vi "StahlPS_Pbus.UpdateOnOff.vi"(0 "i ref in":refnum<vi>, 1 "badValue":bool, 2 "moduleValue":dbl format="%.2f", 3 "ms timeout (10000)":i32=10000, 5 "error in (no error)":errorcluster, 6 "onOffQuality":i32) -> (14 "i ref out":refnum<vi>, 17 "timed out":bool, 19 "error out":errorcluster)   [LabVIEW 2014, in "StahlPS_Pbus.lvlib"]
doc: "Takes the value published by the module and calculates the on-off state.\n\nThe value is written to the attribute data and published via DIM.\n\nThe bad-status bit is also determined and updated."
uses:
  StahlPS_Pbus.lvlib
  CSlibraries/UtilityLib/UtilityLib.valueStatus.ctl
  CSCore/CSApplicationBaseClasses/PSChannelBase/PSChannelBase.statusType.ctl
  CSCore/CSApplicationBaseClasses/PSChannelBase/PSChannelBase.directionType.ctl
  CSCore/CSApplicationBaseClasses/PSChannelBase/PSChannelBase.serviceType.ctl
  CSCore/CSApplicationBaseClasses/DeviceBase/DeviceBase.deviceState.ctl
  CSCore/CSApplicationBaseClasses/PSChannelBase/PSChannelBase.lvlib
  CSlibraries/UtilityLib/UtilityLib.lvlib
  CSCore/CSApplicationBaseClasses/DeviceBase/DeviceBase.lvlib
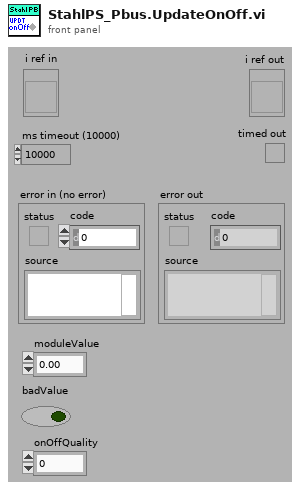
[diagram p1: front panel]
types:
  T1 = typedef "UtilityLib.lvlib/UtilityLib.valueStatus.ctl" = enum16{"no info available", "stand by/off", "on", "warning", "alarm/malfunction", "not implemented", "user action required", "important information", "system default", "control default", "indicator default", "button default"}
  T2 = typedef "PSChannelBase.lvlib/PSChannelBase.serviceType.ctl" = enum16{"onOff", "voltage", "current", "tripCurrent", "rampUpSpeed", "rampDownSpeed", "status"}
  T3 = typedef "DeviceBase.lvlib/DeviceBase.deviceState.ctl" = i16
  T4 = typedef "PSChannelBase.lvlib/PSChannelBase.directionType.ctl" = enum16{"unknown", "update actual value", "update nominal value", "update both"}
  T5 = typedef "PSChannelBase.lvlib/PSChannelBase.statusType.ctl" = i32
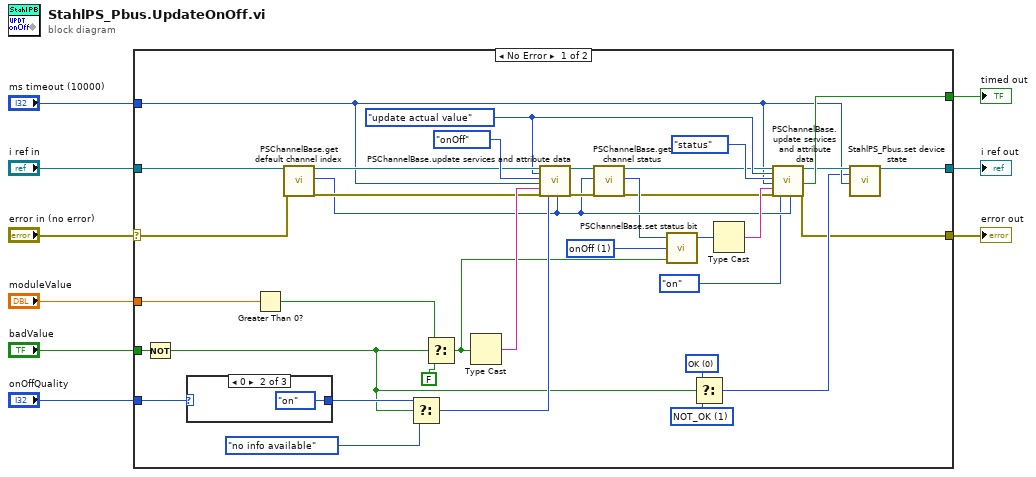
[diagram p0: block diagram]
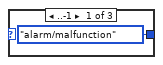
[diagram p2: hidden frame]
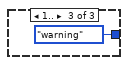
[diagram p3: hidden frame]
diagram:
  n1 = case shown="No Error" "error in (no error)" {
    selector: "error in (no error)" -> [w29 w49]
    tunnel: "i ref in" -> [w30 w50]
    tunnel: "moduleValue" -> [w32 _]
    tunnel: "ms timeout (10000)" -> [w15 _]
    tunnel: [w16 w50] -> w6
    tunnel: [w10 w49] -> w5
    tunnel: [w33 _] -> w4
    tunnel: "badValue" -> [w45 _]
    tunnel: "onOffQuality" -> [w44 _]
    frame No Error {
      w14 = T3 1 items=["ERROR"=-1, "OK"=0, "NOT_OK"=1] ("f")
      w13 = T3 0 items=["ERROR"=-1, "OK"=0, "NOT_OK"=1] ("deviceState")
      w37 = PSChannelBase.directionType."update actual value" ("direction")
      w24 = T5 1 items=["onOff"=1, "inRange"=2, "rampingUp"=4, "rampingDown"=8, "tripped"=16, "error"=32] ("service")
      n2 = Not(x=w45) -> (.not. x?=w12:bool)
      n3 = case shown="0" w44 {
        tunnel: [UtilityLib.valueStatus."alarm/malfunction" ("quality") UtilityLib.valueStatus."on" ("quality") UtilityLib.valueStatus."warning" ("quality")] -> w43
        frame ..-1 {
        }
        frame 0 {
        }
        frame 1.. {
        }
      }
      n4 = Greater Than 0?(x=w32) -> (x > 0?=w23:bool)
      n5 = call "PSChannelBase.get default channel index.vi"("i ref in"=w30, "error in (no error)"=w29) -> ("i ref out"=w39:refnum<vi>, "defaultChannelIndex"=w26:i32, "error out"=w38:errorcluster)  [unwired: 15 in]
      n6 = Select(t=w43, s=w12, f=UtilityLib.valueStatus."no info available" ("quality")) -> (s? t:f=w35:T1)
      n7 = Select(t=w23, s=w12, f=FALSE) -> (s? t:f=w18:bool)
      n8 = Type Cast(x=w18) -> (*(type *) &x=w40:string)  [unwired: 1 in]
      n9 = call "PSChannelBase.update services and attribute data.vi"("i ref in"=w39, "direction"=w37, "service"=PSChannelBase.serviceType."onOff", "ms timeout (10000)"=w15, "value"=w40, "error in (no error)"=w38, "quality"=w35, "channelNumber"=w26) -> ("i ref out"=w28:refnum<vi>, "error out"=w27:errorcluster)  [unwired: 9 in, 1 out]
      n10 = call "PSChannelBase.get channel status.vi"("i ref in"=w28, "channelIndex"=w26, "error in (no error)"=w27) -> ("i ref out"=w20:refnum<vi>, "status"=w25:i32, "error out"=w19:errorcluster)  [unwired: 14 in]
      n11 = call "PSChannelBase.set status bit.vi"("set"=w18, "statusBit"=w24, "status"=w25) -> ("status out"=w22:T5)  [unwired: 2 in]
      n12 = Select(t=w13, s=w12, f=w14) -> (s? t:f=w11:T3)
      n13 = Type Cast(x=w22) -> (*(type *) &x=w34:string)  [unwired: 1 in]
      n14 = call "PSChannelBase.update services and attribute data.vi"("i ref in"=w20, "direction"=w37, "service"=PSChannelBase.serviceType."status", "ms timeout (10000)"=w15, "value"=w34, "error in (no error)"=w19, "quality"=UtilityLib.valueStatus."on", "channelNumber"=w26) -> ("i ref out"=w17:refnum<vi>, "timed out"=w33:bool, "error out"=w10:errorcluster)  [unwired: 9 in]
      n15 = call "StahlPS_Pbus.set device state.vi"("i ref in"=w17, "deviceState"=w11, "ms timeout (10000)"=w15) -> ("i ref out"=w16:refnum<vi>)  [unwired: 14 in, 2 out]
    }
    frame Error {
    }
  }
  "error out" <- w5
  "i ref out" <- w6
  "timed out" <- w4
